vi "Read Timeout [ms].vi"(8 "error in (no error)":errorcluster, 11 "IEventHandler in":refnum<class "IEventHandler.lvclass">) -> (0 "error out":errorcluster, 2 "Timeout [ms]":i32=-1, 3 "IEventHandler out":refnum<class "IEventHandler.lvclass">)   [LabVIEW 2019, in "ActorEvents.lvlib" / "IEventHandler.lvclass"]
uses:
  <vilib>/gpm_packages/@cs/mva-viewable/Source/ActorEvents/IEventHandler/IEventHandler.lvclass
  <vilib>/gpm_packages/@cs/mva-viewable/Source/ActorEvents/IEventHandler/IEventHandler.lvclass/IEventHandler.ctl
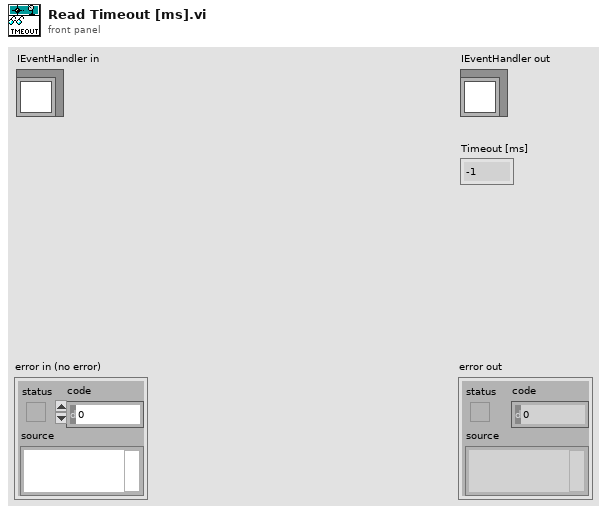
[diagram p1: front panel]
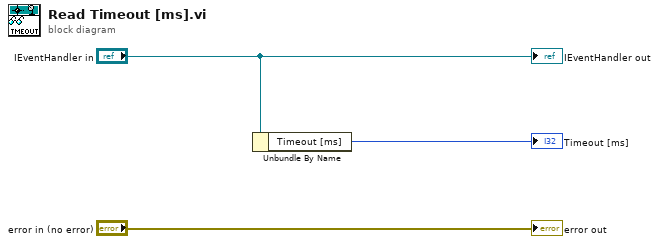
[diagram p0: block diagram]
diagram:
  n1 = Unbundle By Name("IEventHandler in") -> ("Timeout [ms]"=→"Timeout [ms]":i32)
  "error out" <- "error in (no error)"
  "IEventHandler out" <- "IEventHandler in"
